vi "Check Angle.vi"(11 "Input String Read Angle":string) -> (3 "Mirror Angle":dbl, 4 "error out":errorcluster)   [LabVIEW 2020, in "FBN_LATM.lvlib"]
uses:
  FBN_LATM.lvlib
  <vilib>/regexp/Match Regular Expression.xnode
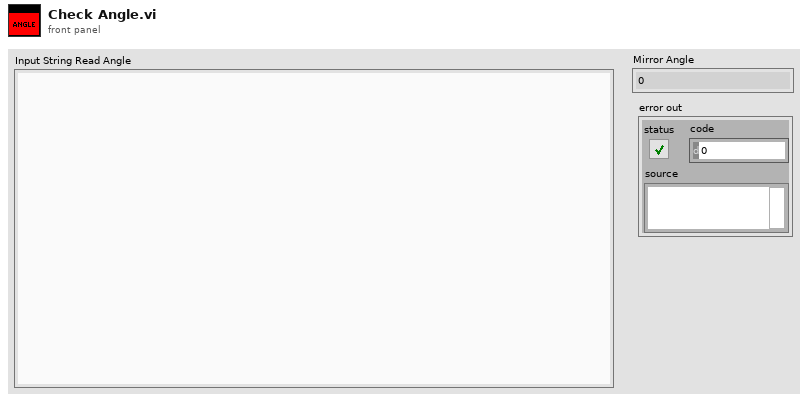
[diagram p1: front panel]
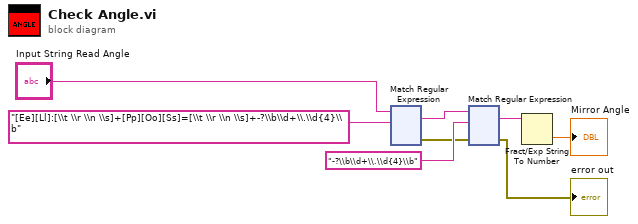
[diagram p0: block diagram]
diagram:
  n1 = xnode "Match Regular Expression"("input string"="Input String Read Angle", "regular expression"="[Ee][Ll]:[\\t \\r \\n \\s]+[Pp][Oo][Ss]=[\\t \\r \\n \\s]+-?\\b\\d+\\.\\d{4}\\b") -> ("whole match"=w6:string, "error out"=w2:errorcluster)  [unwired: 4 in, 3 out]
  n2 = xnode "Match Regular Expression"("input string"=w6, "regular expression"="-?\\b\\d+\\.\\d{4}\\b", "error in"=w2) -> ("whole match"=w4:string, "error out"=→"error out":errorcluster)  [unwired: 3 in, 3 out]
  n3 = Fract/Exp String To Number(string=w4) -> (number=→"Mirror Angle":dbl)  [unwired: 3 in, 1 out]
